vi "Temperature Limit.vi"() -> ()   [LabVIEW 2012]
doc: "该VI可仿真温度采集，绘制温度图形，并通知用户温度是否超出范围。"
panel:
  in  "开始":bool
  in  "△t(ms)":i32(slide)=400 scale=50.0..500.0
  in  "停止":bool
  in  "上限":dbl=28.0 format="%.2f"
  out "温度":cluster{"Temperature":dbl, "High Limit":dbl}(graph)={"Temperature"=85.88749999999999, "High Limit"=80.0}
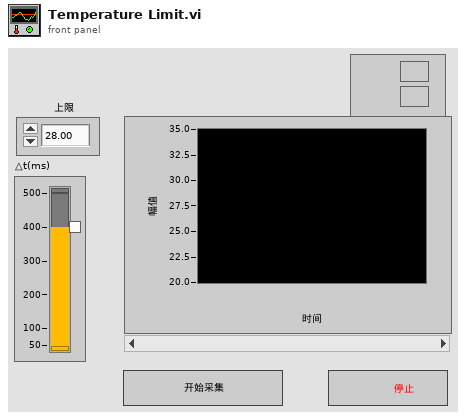
[diagram p1: front panel]
types:
  T1 = enum16{"Always On", "Always Off", "Off While Running"}
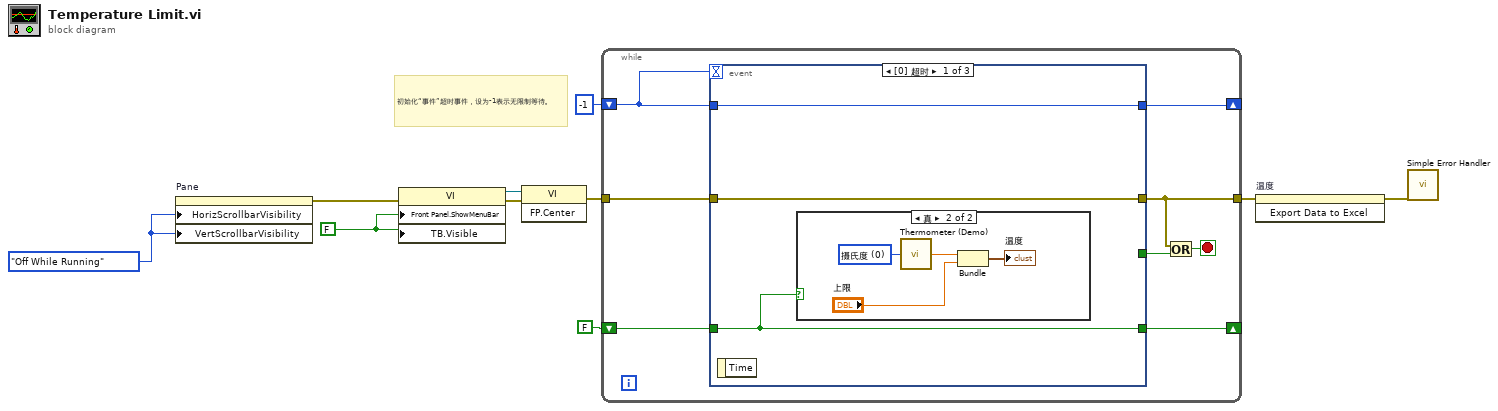
[diagram p0: block diagram]
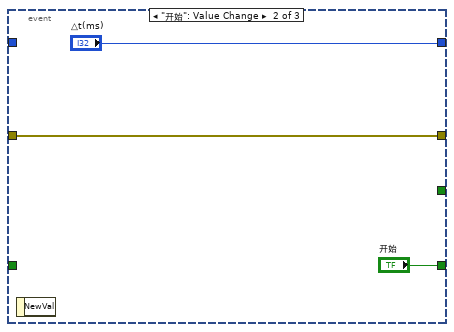
[diagram p3: hidden frame]
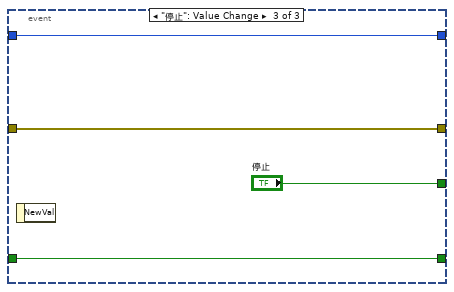
[diagram p4: hidden frame]
diagram:
  w5 = T1."Off While Running" ("水平滚动条可见")
  w8 = FALSE
  # "初始化“事件”超时事件，设为-1表示无限制等待。"
  n1 = property on="Pane" class="Pane"("HorizScrollbarVisibility"=w5, "VertScrollbarVisibility"=w5) -> (error out=w4:errorcluster)  [unwired: 2 in, 1 out]
  n2 = property on="属性节点" class="VI"(error in=w4, "Front Panel.ShowMenuBar"=w8, "TB.Visible"=w8) -> (reference out=w7:refnum<vi>, error out=w6:errorcluster)  [unwired: 1 in]
  n3 = invoke on="调用节点" class="VI" method="FP.Center"(reference=w7, error in=w6) -> (error out=w3:errorcluster)  [unwired: 1 in, 2 out]
  n4 = while {
    tunnel: w3 -> [w18]
    tunnel: [w16] -> w2
    shift-right: [w14] -> _
    shift-left: FALSE ("开始") -> [w13]
    shift-right: [w12] -> _
    shift-left: -1 ("△t(ms)") -> [w11]
    stop <- w17 stop-if-true
    n5 = event shown="[0] 超时" {
      selector: _ -> [_ _ _]
      dyn-events: _ -> [_ _ _]
      timeout: w11 -> [_ _ _]
      tunnel: [_ _ "停止"] -> w15
      tunnel: w18 -> [w21 w26 w31]
      tunnel: [w21 w26 w31] -> w16
      tunnel: [w19 "开始" w30] -> w14
      tunnel: w13 -> [w19 _ w30]
      tunnel: [w20 "△t(ms)" w29] -> w12
      tunnel: w11 -> [w20 _ w29]
      event Timeout {
        n6 = event-data ("事件数据节点")() -> ()  [unwired: 1 in, 1 out]
        n7 = case shown="真" w19 {
          frame False {
          }
          frame True {
            w22 = u16 0 items=["摄氏度", "华氏度"] ("单位（0：摄氏度）")
            n8 = call "Thermometer (Demo).vi"("单位（0：摄氏度）"=w22) -> ("温度值"=w23:dbl)
            n9 = Bundle ("捆绑")("温度值"=w23, "上限"="上限") -> (→"温度":cluster{"温度值":dbl, "上限":dbl})  [unwired: 1 in]
          }
        }
      }
      event "开始": Value Change {
        n10 = event-data ("事件数据节点")() -> ()  [unwired: 1 in, 1 out]
      }
      event "停止": Value Change {
        n11 = event-data ("事件数据节点")() -> ()  [unwired: 1 in, 1 out]
      }
    }
    n12 = Or ("或")(x=w16, y=w15) -> (x .or. y?=w17:bool)
  }
  n13 = invoke on="温度" class="WFChart (strict)" method="Export Data to Excel"(error in=w2) -> (error out=w1:errorcluster)  [unwired: 2 in, 2 out]
  n14 = call <vilib>:"Simple Error Handler.vi"("error in (no error)"=w1) -> ()  [unwired: 4 in, 5 out]
